vi "Encorder.vi"(7 "error in (no error)":errorcluster, 8 "Reset Counter":bool, 10 "Enum":enum16{"M4", "M3", "M2", "M1"}(ring)) -> (0 "error out":errorcluster, 3 "en/deg":dbl)   [LabVIEW 2018]
uses:
  <vilib>/myRIO/Common/Instrument Driver Framework/myRIO v1.0/Encoder/typedefs/Encoder Count Direction Enum.ctl
  <vilib>/myRIO/Common/Instrument Driver Framework/myRIO v1.0/Encoder/typedefs/Encoder Signal Mode.ctl
  <vilib>/Utility/error.llb/Error Cluster From Error Code.vi
  <vilib>/myRIO/Common/Instrument Driver Framework/myRIO v1.0/Encoder/vis/myRIO v1.0 Read Encoder.vi
  <vilib>/myRIO/Instrument Drivers/Onboard IO/Encoder/Encoder.lvlib
panel:
  out "Overflow?":bool
  out "Counter Direction":T1
  out "Counter Value":i32
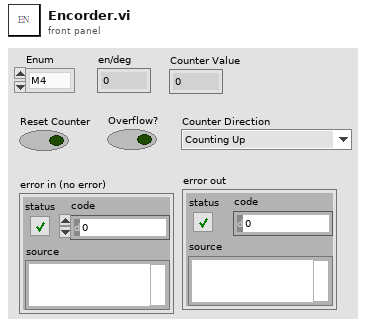
[diagram p1: front panel]
types:
  T1 = typedef "Encoder Count Direction Enum.ctl" = enum16{"Counting Up", "Counting Down"}
  T2 = typedef "Encoder Signal Mode.ctl" = enum16{"Quadrature phase signal", "Step and direction signal"}
  T3 = typedef "Encoder.lvlib/Encoder Reference.ctl" = cluster{"myRIO Reference":T4, "Encoder Channels Enum":T8}
  T4 = typedef "myRIO Generic Hardware Reference.ctl" = cluster{"myRIO Model":T5, "myRIO Hardware Reference":T6}
  T5 = typedef "Hardware Version Enum.ctl" = enum16{"Unknown", "myRIO-1900", "myRIO-1950", "roboRIO", "NI ELVIS RIO CM", "ELVIS III"}
  T6 = typedef "myRIO v1.0 Reference.ctl" = cluster{"Generic FPGA Reference":T7, "Allow multiple opens":bool}
  T7 = typedef "Generic FPGA Reference.ctl" = refnum<k20>
  T8 = typedef "Encoder Channels Enum.ctl" = enum16{"Not Connected", "C/ENC0", "C/ENC1", "A/ENC", "A/ENC0", "A/ENC1", "A/ENC2", "A/ENC3", "A/ENC4", "A/ENC5", "A/ENC6", "A/ENC7", "A/ENC8", "A/ENC9", "B/ENC", "B/ENC0", "B/ENC1", "B/ENC2", "B/ENC3", "B/ENC4", "B/ENC5", "B/ENC6", "B/ENC7", "B/ENC8", "B/ENC9", "DIO/ENC0", "DIO/ENC1", "DIO/ENC2", "DIO/ENC3", "DIO/ENC4"}
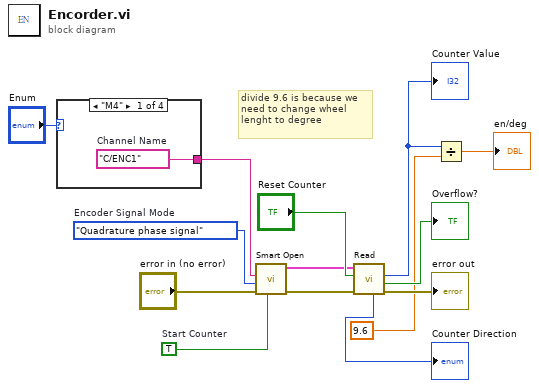
[diagram p0: block diagram]
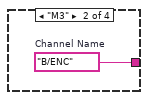
[diagram p2: hidden frame]
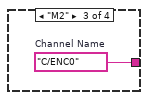
[diagram p3: hidden frame]
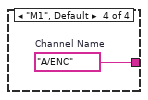
[diagram p4: hidden frame]
diagram:
  w13 = TRUE  # Start Counter
  w14 = Encoder_Signal_Mode."Quadrature phase signal"  # Encoder Signal Mode
  # "divide 9.6 is because we need to change wheel lenght to degree"
  n1 = case shown="\"M4\"" "Enum" {
    tunnel: [w15 w16 w17 w18] -> w5
    frame "M4" {
      w15 = tag "C/ENC1"  # Channel Name
    }
    frame "M3" {
      w16 = tag "B/ENC"  # Channel Name
    }
    frame "M2" {
      w17 = tag "C/ENC0"  # Channel Name
    }
    frame "M1", Default {
      w18 = tag "A/ENC"  # Channel Name
    }
  }
  n2 = call <vilib>:"Smart Open.vi"("Start Counter"=w13, "error in (no error)"="error in (no error)", "Encoder Signal Mode"=w14, "Channel Name"=w5) -> ("error out"=w8:errorcluster, "Encoder Ref Out"=w9:T3)  [unwired: 6 in]
  n3 = call <vilib>:"Read.vi"("error in (no error)"=w8, "Reset Counter"="Reset Counter", "Encoder Ref In"=w9) -> ("error out"=→"error out":errorcluster, "Overflow?"=→"Overflow?":bool, "Counter Value"=w1:i32, "Counter Direction"=→"Counter Direction":T1)  [unwired: 4 in, 1 out]
  "Counter Value" <- w1
  n4 = Divide(x=w1, y=9.6) -> (x/y=→"en/deg":dbl)
